vi "Close Property.vi"(0 "SLSC Remote in":refnum<class "SLSC Remote.lvclass">, 5 "property":refnum<k21>, 11 "error in (no error)":errorcluster) -> (4 "SLSC Remote out":refnum<class "SLSC Remote.lvclass">, 15 "error out":errorcluster)   [LabVIEW 2015, in "SLSC Remote.lvclass"]
uses:
  SLSC Remote.lvclass
  <vilib>/NI/i3 JSON/JSON Generation/Create Value Files/Create Value - Object.vi
  <vilib>/NI/i3 JSON/JSON Generation/Add Object Parameter Files/Add Object Parameter - String.vi
  <vilib>/NI/NI JSONRPC Server Framework/Classes/Server/Format Client Request (Auto-Increment).vi
  <vilib>/httpClient/POSTBuffer.vi
  <vilib>/NI/NI JSONRPC Server Framework/Classes/Server/JSONRPC Server.lvclass
  <vilib>/NI/i3 JSON/i3-json.lvlib
  <vilib>/httpClient/LabVIEWHTTPClient.lvlib
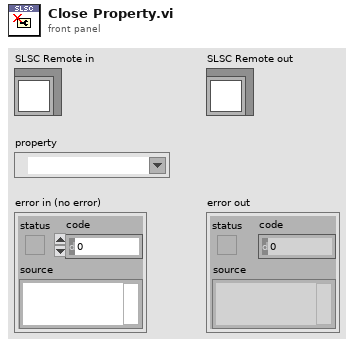
[diagram p1: front panel]
types:
  T1 = typedef "LabVIEWHTTPClient.lvlib/ClientHandle.ctl" = refnum<k1>
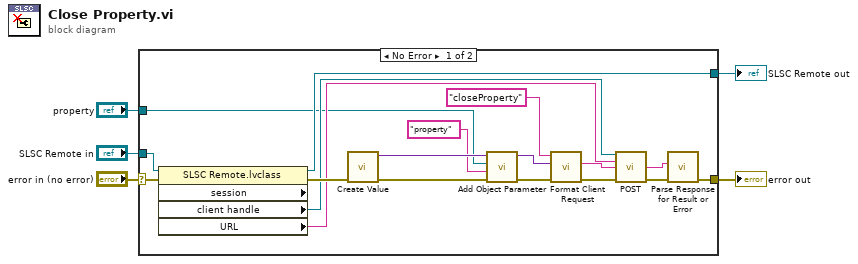
[diagram p0: block diagram]
diagram:
  n1 = case shown="No Error" "error in (no error)" {
    selector: "error in (no error)" -> [w20 w24]
    tunnel: "SLSC Remote in" -> [w22 w25]
    tunnel: [w21 w25] -> w1
    tunnel: [w10 w24] -> w2
    tunnel: "property" -> [w9 _]
    frame No Error {
      n2 = property class="SLSC Remote.lvclass" props=["session", "client handle", "URL"](reference=w22, error in=w20) -> (reference out=w21:refnum<class "SLSC Remote.lvclass">, error out=w19:errorcluster, "client handle"=w15:T1, "URL"=w14:string)  [unwired: 1 out]
      n3 = call-poly <vilib>:"Create Value.vi"("error in (no error)"=w19) -> ("error out"=w18:errorcluster, "JSON Tree"=w23:variant)  [unwired: 9 in]
      n4 = call-poly <vilib>:"Add Object Parameter.vi"("error in (no error)"=w18, "Name"="property", "String"=w9, "JSON Tree in (JSON Object)"=w23) -> ("error out"=w6:errorcluster, "JSON Tree out (JSON Object)"=w7:variant)  [unwired: 6 in]
      n5 = call-poly <vilib>:"Format Client Request.vi"("error in (no error)"=w6, "params"=w7, "method"="closeProperty") -> ("error out"=w13:errorcluster, "Request String"=w16:string)  [unwired: 7 in]
      n6 = call-poly <vilib>:"POST.vi"("client handle"=w15, "url"=w14, "buffer"=w16, "error in (no error)"=w13) -> ("body"=w12:string, "error out"=w11:errorcluster)  [unwired: 8 in, 2 out]
      n7 = call <vilib>:"Parse Response for Result or Error.vi"("error in"=w11, "Response String In"=w12) -> ("error out"=w10:errorcluster)  [unwired: 7 in, 2 out]
    }
    frame Error {
    }
  }
  "error out" <- w2
  "SLSC Remote out" <- w1
